vi "Configure Channel.vi"   [LabVIEW 2009, in "MicroDAQ.lvlib"]
doc: "This VI configures task settings. This VI is polimorphic and will adapt to source from Create channel.VI."
uses:
  <instrlib>/MicroDAQ/MicroDAQ.lvlib
  <instrlib>/MicroDAQ/Channel/Analog Output/Analog output.lvclass
  <instrlib>/MicroDAQ/Channel/Analog Input/Analog Input.lvclass
  <instrlib>/MicroDAQ/Channel/PWM/PWM.lvclass
  <instrlib>/MicroDAQ/Channel/DSP/DSP.lvclass
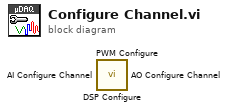
[diagram p0: block diagram]
diagram:
  n1 = call <instrlib>:"DSP Configure.vi"() -> ()  [unwired: 10 in, 2 out]
  n2 = call <instrlib>:"PWM Configure.vi"() -> ()  [unwired: 10 in, 2 out]
  n3 = call <instrlib>:"AI Configure Channel.vi"() -> ()  [unwired: 10 in, 2 out]
  n4 = call <instrlib>:"AO Configure Channel.vi"() -> ()  [unwired: 10 in, 2 out]
